vi "TCP Send Info.vi"(8 "error in (no error)":errorcluster, 10 "data in":string, 11 "TCP Network Connection in":T1) -> (0 "error out":errorcluster, 3 "TCP Network Connection out":T1)   [LabVIEW 2020, in "CSM-TCP-Router.lvlib"]
uses:
  CSM-TCP-Router.lvlib
  <vilib>/addons/_JKI.lib/_JKI_lib_TCP_Server.llb/TCP Server Connection Session ID Cluster.ctl
  tcp-msg type.ctl
  <vilib>/addons/_JKI.lib/_JKI_lib_TCP_Server.llb/JKI TCP Server.lvclass
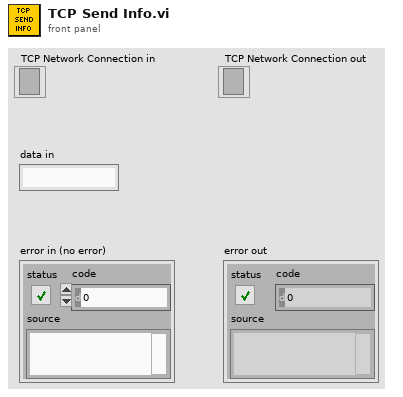
[diagram p1: front panel]
types:
  T1 = typedef "JKI TCP Server.lvclass/TCP Server Connection Session ID Cluster.ctl" = refnum<k5>
  T2 = typedef "CSM-TCP-Router.lvlib/tcp-msg type.ctl" = enum8{"info", "error", "cmd", "cmd-resp", "resp", "async-resp", "status", "interrupt"}
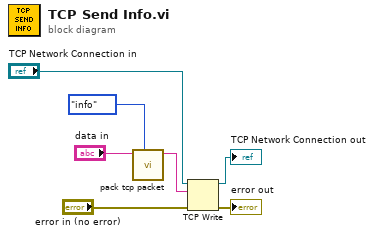
[diagram p0: block diagram]
diagram:
  n1 = call "pack tcp packet.vi"("tcp-message-type"=tcp-msg_type."info", "String"="data in") -> ("TCP Pack"=w6:string)  [unwired: 9 in]
  n2 = TCP Write(connection ID="TCP Network Connection in", data in=w6, error in (no error)="error in (no error)") -> (connection ID out=→"TCP Network Connection out":T1, error out=→"error out":errorcluster)  [unwired: 1 in, 1 out]
